vi "LJStreamM build log header string.vi"(1 "Names":string[](array[string]), 2 "# Channels":i32) -> (0 "Header String":string)   [LabVIEW 2026]
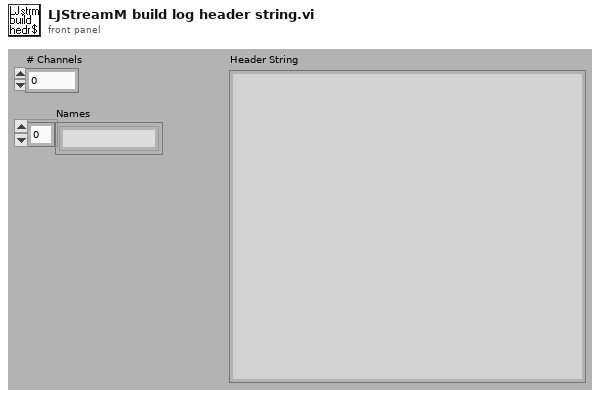
[diagram p1: front panel]
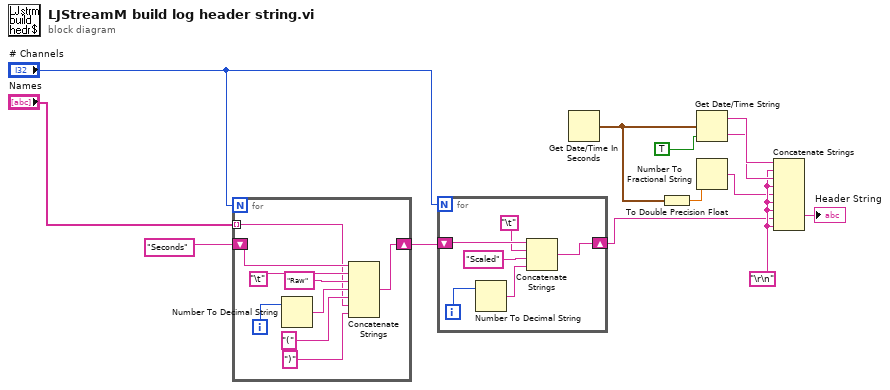
[diagram p0: block diagram]
diagram:
  w8 = "\r\n"
  n1 = for {
    N: "# Channels" -> [_]
    shift-right: [w21] -> w4
    shift-left: "Seconds" ("Substring") -> [w22]
    tunnel: "Names" -> [w15] mode=indexing
    i -> [w19]
    n2 = Number To Decimal String(number=w19) -> (decimal integer string=w18:string)  [unwired: 1 in]
    n3 = Concatenate Strings(w22, "\t", "Raw" ("string"), w18, "(" ("string"), w15, ")" ("Substring")) -> (w21:string)
  }
  n4 = for {
    N: "# Channels" -> [_]
    shift-right: [w27] -> w3
    shift-left: w4 -> [w28]
    i -> [w24]
    n5 = Number To Decimal String(number=w24) -> (decimal integer string=w23:string)  [unwired: 1 in]
    n6 = Concatenate Strings(w28, "\t", "Scaled" ("Substring"), w23) -> (w27:string)
  }
  n7 = Get Date/Time In Seconds() -> (seconds since 1Jan1904=w6:timestamp)
  n8 = To Double Precision Float(number=w6) -> (double precision float=w9:dbl)
  n9 = Get Date/Time String(seconds (now)=w6, want seconds? (F)=TRUE) -> (date string=w13:string, time string=w12:string)  [unwired: 1 in]
  n10 = Number To Fractional String(number=w9) -> (F-format string=w7:string)  [unwired: 3 in]
  n11 = Concatenate Strings(w13, w8, w12, w8, w7, w8, w8, w3, w8) -> (→"Header String":string)
